vi "CAlex2_rtDisplay_Scale.vi"(1 "Scale (1) and Offset (0,0)":cluster{"x":i16, "y":i16, "Scale":dbl}={"x"=0, "y"=0, "Scale"=1.0}, 3 "Input XYZ array":dbl[][](array[numeric])) -> (0 "Output XY array":cluster{i16, i16}[](array[cluster]))   [LabVIEW 2016, in "CAlex2.lvclass"]
uses:
  CAlex2/CAlex2.lvclass
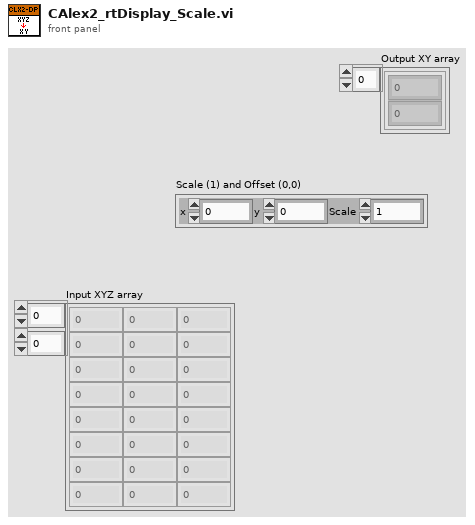
[diagram p1: front panel]
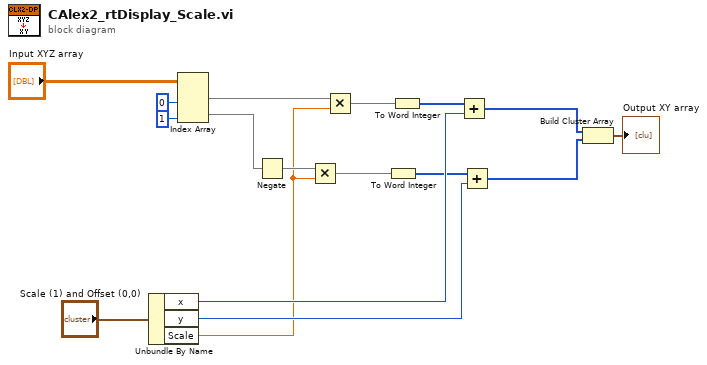
[diagram p0: block diagram]
diagram:
  n1 = Unbundle By Name("Scale (1) and Offset (0,0)") -> ("x"=w15:i16, "y"=w14:i16, "Scale"=w12:dbl)
  n2 = Index Array(array="Input XYZ array", index (col) #1=0 ("disabled index (col)"), index (col) #2=1 ("index (col)")) -> (element #1=w6:dbl[], element #2=w5:dbl[])  [unwired: 2 in]
  n3 = Negate(x=w5) -> (-x=w13:dbl[])
  n4 = Multiply(x=w13, y=w12) -> (x*y=w2:dbl[])
  n5 = Multiply(x=w6, y=w12) -> (x*y=w4:dbl[])
  n6 = To Word Integer(number=w2) -> (16bit integer=w1:i16[])
  n7 = To Word Integer(number=w4) -> (16bit integer=w3:i16[])
  n8 = Add(x=w3, y=w15) -> (x+y=w7:i16[])
  n9 = Add(x=w1, y=w14) -> (x+y=w11:i16[])
  n10 = Build Cluster Array(w7, w11) -> (→"Output XY array":cluster{i16, i16}[])
